vi "FRIC_navX_Internal_USB_ProcessingLoop.vi"(7 "Device Number":T3, 10 "Serial Port":T2=enum."USB 1", 11 "Rate (4Hz-200Hz)":u8=50 min=4 max=200) -> ()   [LabVIEW 2016]
doc: "This navX VI handles the reading/writing for the navX. All of the good stuff is in here.\nTHIS VI SHOULD NOT BE CALLED BY THE USER!"
uses:
  <vilib>/Rock Robotics/SystemInterfaces/i2clib/i2c_bus.ctl
  TypeDefs/Z900_navX_ProtocolTypeDef.ctl
  navX Library v2.lvlib
  TypeDefs/FRIC_navX_ProcessingLoopStatesTypeDef_I2C.ctl
  TypeDefs/Z900_navX_IntegrationControlRegisters.ctl
  TypeDefs/Z900_navX_ActionTypeDef.ctl
  TypeDefs/Z900_navX_NotifyPacketTypeDef.ctl
  TypeDefs/FRIC_navX_I2C Process Loop TypeDef.ctl
  <vilib>/Rock Robotics/SystemInterfaces/spilib/spi_bus.ctl
  <vilib>/Rock Robotics/WPI/SPI/WPI_SPIDevRef.ctl
  TypeDefs/Z900_navX_SerialStreamTypeDef.ctl
  <vilib>/Rock Robotics/WPI/SerialPort/WPI_SerialPortRef.ctl
  TypeDefs/FRIC_navX_DeviceNumbersTypeDef.ctl
  <vilib>/Rock Robotics/WPI/SerialPort/WPI_SerialPort.ctl
  <vilib>/Platform/TimedLoop/XDataNode/wakeup.ctl
  <vilib>/Platform/TimedLoop/XDataNode/XDNodeRunTimeDep.lvlib
  <vilib>/Platform/TimedLoop/XDataNode/nitl_modes.ctl
  <vilib>/Platform/TimedLoop/XDataNode/timing_clust.ctl
  <vilib>/Platform/TimedLoop/XDataNode/XDataNode.xnode
  <vilib>/ptbypt/NI_PtbyPt.lvlib
  TypeDefs/Z900_navX_DeviceTypeDef.ctl
panel:
  in  "Tab Control":enum32{"Page 1", "Page 2"}(tab)
  in  "Halt":bool
  out "Connected 2":bool
  out "error":errorcluster
  in  "Stream Type":T1=enum."AHRSAndPositioning"
  out "Loop Time":dbl format="%#.1g"
  out "Loop dt":i64
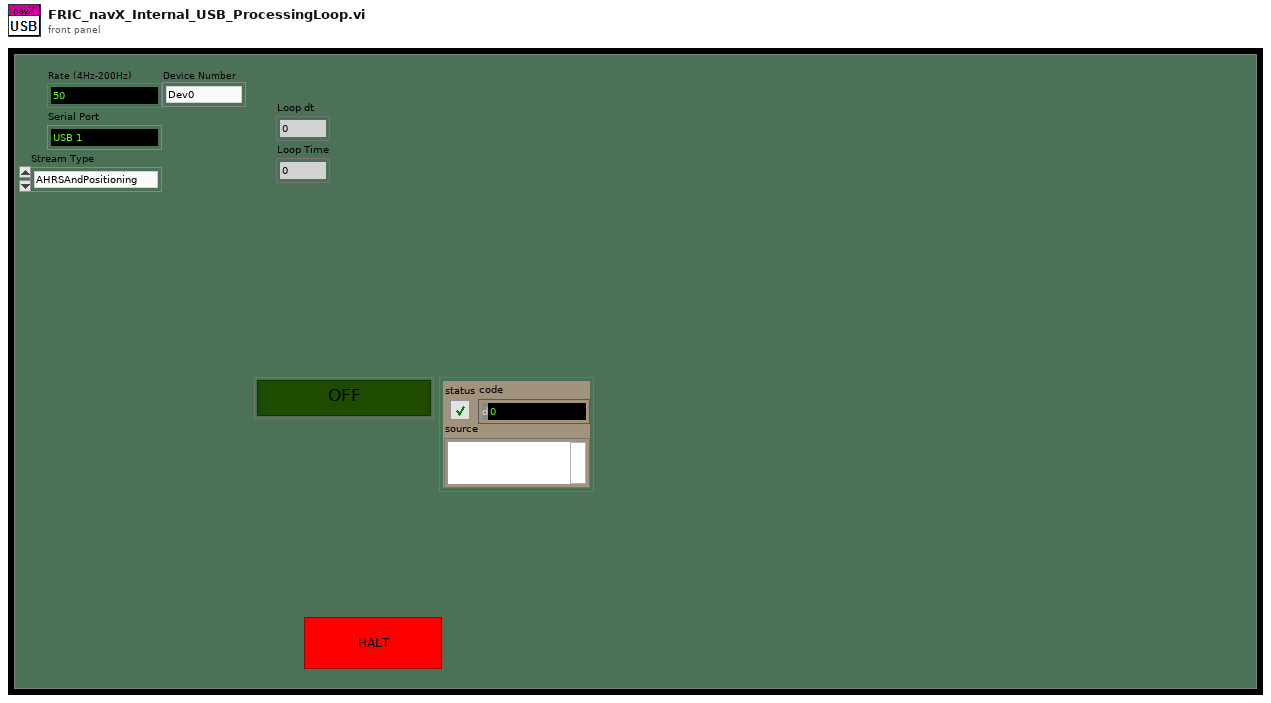
[diagram p1: front panel]
types:
  T1 = typedef "navX Library v2.lvlib/Z900_navX_SerialStreamTypeDef.ctl" = enum16{"YRPH", "Quaterinons", "Gyro/Raw", "AHRS", "AHRSAndPositioning"}
  T2 = typedef "WPI_SerialPort.ctl" = enum16{"Onboard RS-232", "MXP TTL", "USB 1", "USB 2"}
  T3 = typedef "FRIC_navX_DeviceNumbersTypeDef.ctl" = enum16{"Dev0", "Dev1", "Dev2", "Dev3"}
  T4 = typedef "FRIC_navX_I2C Process Loop TypeDef.ctl" = cluster{"State Array":T5[], "error":errorcluster, "FPGA Cluster":cluster{"Last Valid FPGA Time":dbl, "Error Count":i32, "Initialized":bool}, "Device Info":T6, "I2CDevRef":cluster{"DevStatus":errorcluster, "Device Address":u8, "Handle":i32, "I2C Bus":T8}, "Registry":u8[], "Command Array":T9[], "Connected?":bool, "navX Device Memory Size":i32, "notification":T10, "Memory Size Set":bool, "SPIDevRef":T12, "navX Serial Open":cluster{"Stream Type":T1, "Serial Port":T2}, "SerialPortRef":T14, "Serial Read Buffer":string, "Serial Write Buffer":string[], "Device Number":T3, "navX SPI Open":cluster{"SPI Bus":T13, "Clock Rate (Hz)":dbl}, "Loop dt":i64, "current time":timestamp, "Loop Time":i64}
  T5 = typedef "FRIC_navX_ProcessingLoopStatesTypeDef_I2C.ctl" = enum16{"Process", "INI", "Check Packets Valid", "Close", "Flush Serial", "Generate Command", "Last Packet Valid", "Open", "Read", "Reset Serial", "Set Termination Char", "Update AE", "Wait", "Write", "Exit"}
  T6 = typedef "navX Library v2.lvlib/Z900_navX_DeviceTypeDef.ctl" = cluster{"Interface":cluster{"Protocol":T7, "Update Rate (4Hz-100Hz)":u8, "navX Open TypeDef":variant}, "Notify Packet":refnum<notifier>, "Loop VI Refnum":refnum<vi>, "Ready to Close Occurrence Refnum":refnum<k4>}
  T7 = typedef "navX Library v2.lvlib/Z900_navX_ProtocolTypeDef.ctl" = enum16{"SERIAL", "I2C", "SPI"}
  T8 = typedef "i2c_bus.ctl" = enum16{"I2C On-Board", "I2C MXP", "Invalid"}
  T9 = typedef "navX Library v2.lvlib/Z900_navX_IntegrationControlRegisters.ctl" = u8
  T10 = typedef "navX Library v2.lvlib/Z900_navX_NotifyPacketTypeDef.ctl" = cluster{"navX Action":T11, "Data":variant}
  T11 = typedef "navX Library v2.lvlib/Z900_navX_ActionTypeDef.ctl" = enum16{"None", "Halt", "Update Serial Protocol", "Zero-Yaw", "Zero-Displacement", "Zero-Velocity"}
  T12 = typedef "WPI_SPIDevRef.ctl" = cluster{"DevStatus":errorcluster, "Handle":i32, "SPI Bus":T13}
  T13 = typedef "spi_bus.ctl" = enum16{"SPI On-Board, CS0", "SPI On-Board, CS1", "SPI On-Board, CS2", "SPI On-Board, CS3", "SPI MXP", "Invalid"}
  T14 = typedef "WPI_SerialPortRef.ctl" = cluster{"DevStatus":errorcluster, "Serial Port Name":refnum<visa-resource-name>}
  T15 = typedef "XDNodeRunTimeDep.lvlib/timing_clust.ctl" = cluster{"Expected End [f-1]":u64, "Actual End [f-1]":u64, "Finished Late? [f-1]":bool, "Expected End [i-1]":u64, "Actual End [i-1]":u64, "Finished Late? [i-1]":bool, "Expected Start [i]":u64, "Actual Start [i]":u64, "Expected Start [f]":u64, "Actual Start [f]":u64, "Source Name":string, "Structure Name":string, "Period":i64, "Deadline":i64, "Offset":i64, "Start":i64, "Priority":i32, "Timeout":i32, "Mode":T16, "Wakeup Reason":T17, "Error":errorcluster, "Source Type":string, "Secondary Source Type":string, "Global End Time":u64, "Global Start Time":u64, "Frame Duration":u64, "Iteration Duration":u64, "Assigned CPU":i32, "I/O Scan Engine Mode":u32}
  T16 = typedef "XDNodeRunTimeDep.lvlib/nitl_modes.ctl" = enum32{"No Change", "Process missed periods, maintain original phase", "Discard missed periods, maintain original phase", "Process missed periods, ignore original phase", "Discard missed periods, ignore original phase"}
  T17 = typedef "XDNodeRunTimeDep.lvlib/wakeup.ctl" = enum32{"Normal", "Aborted", "Asynchronous wakeup", "Timing source error", "Timed loop error", "Timeout"}
  T18 = typedef "Z900_navX_ActionTypeDef.ctl" = enum16{"None", "Halt", "Normal Read", "Update Serial Protocol", "Update Rate Htz", "Zero-Yaw", "Zero-Displacement", "Zero-Velocity"}
  T19 = cluster{"Last Valid FPGA Time":dbl, "Error Count":i32, "Initialized":bool}
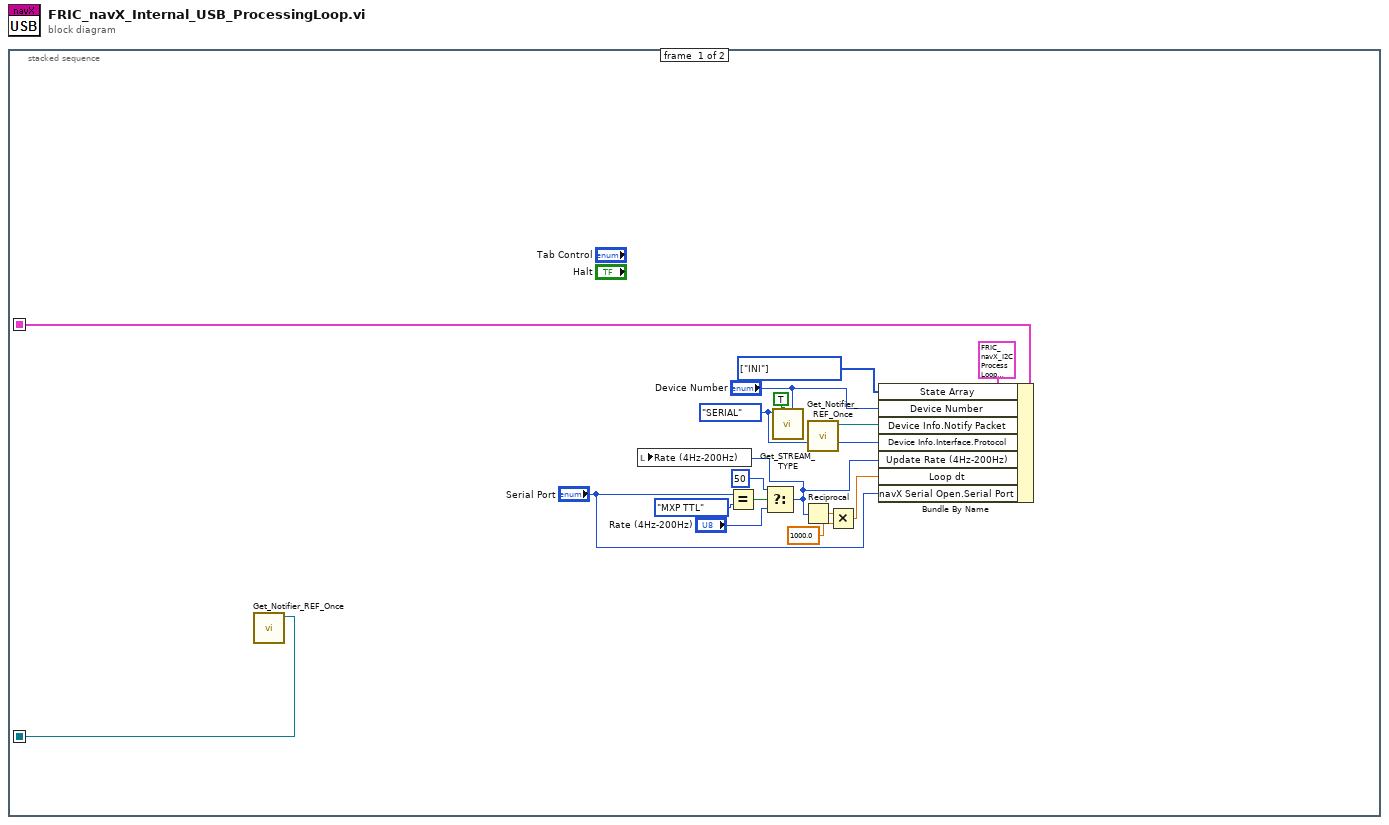
[diagram p0: block diagram]
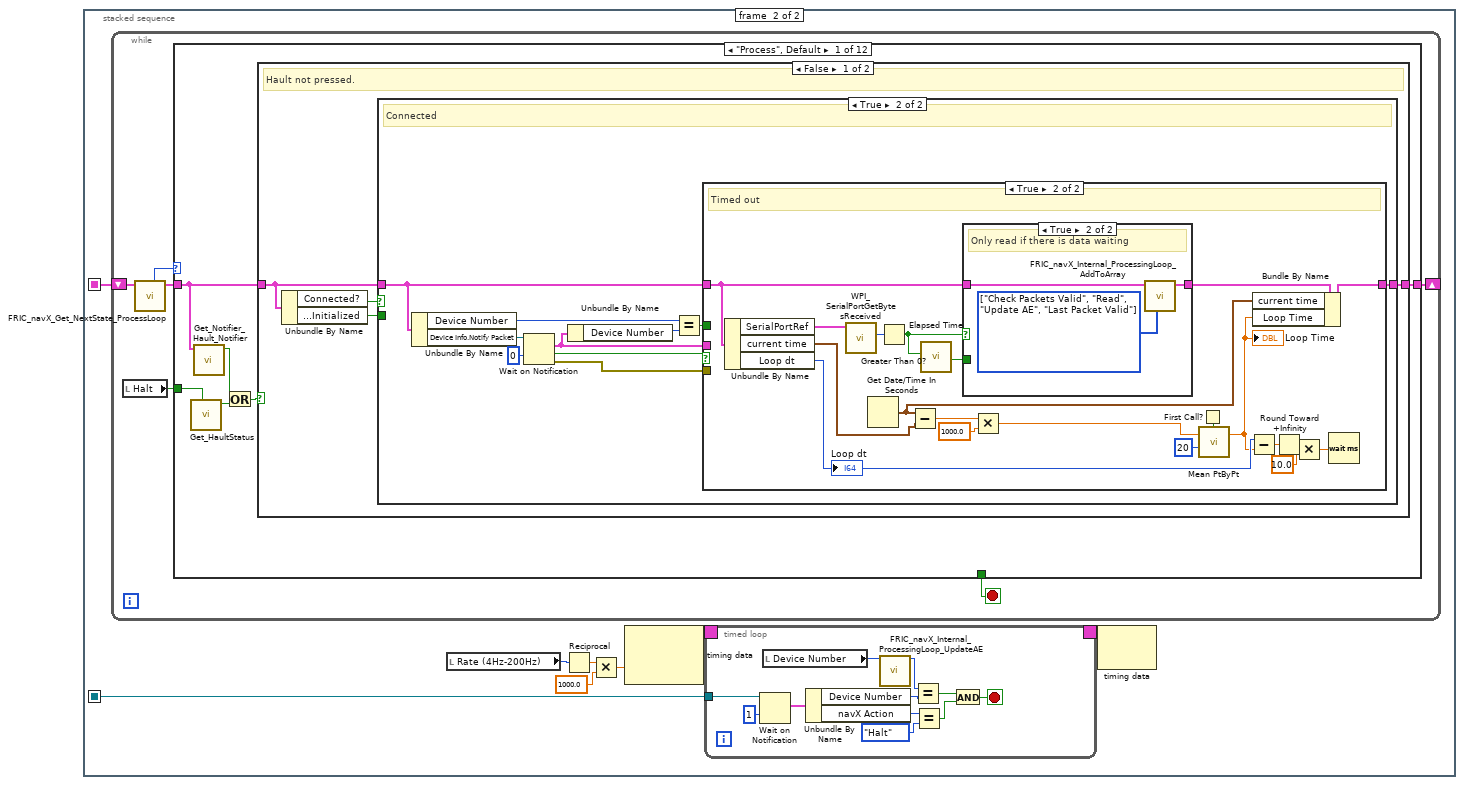
[diagram p2: hidden frame]
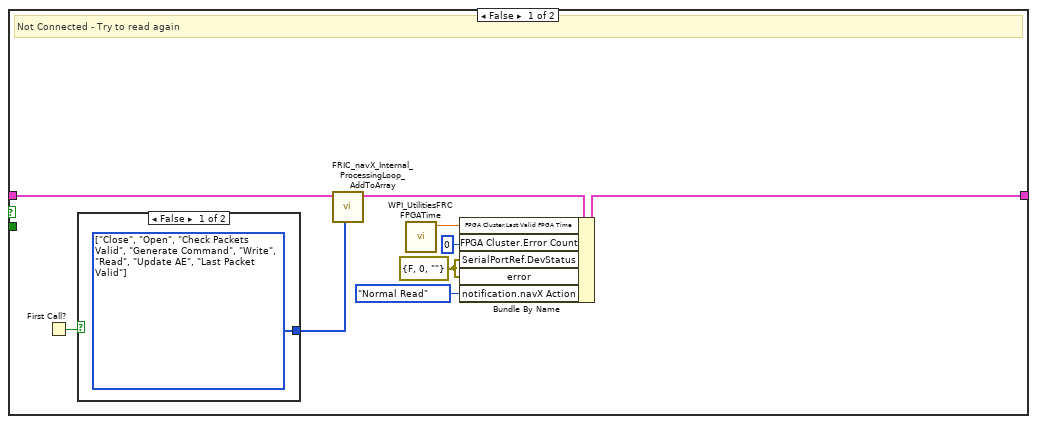
[diagram p3: hidden frame]
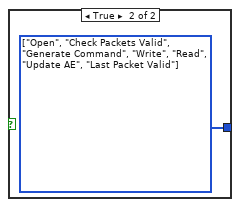
[diagram p4: hidden frame]
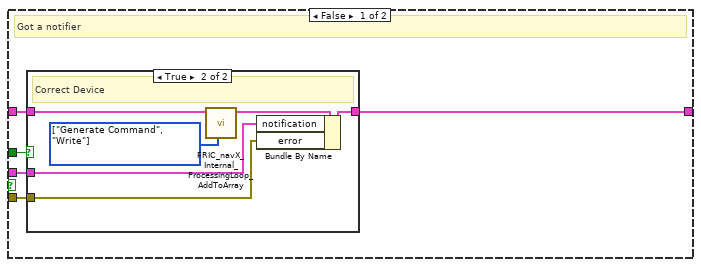
[diagram p5: hidden frame]
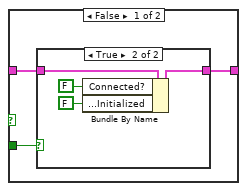
[diagram p7: hidden frame]
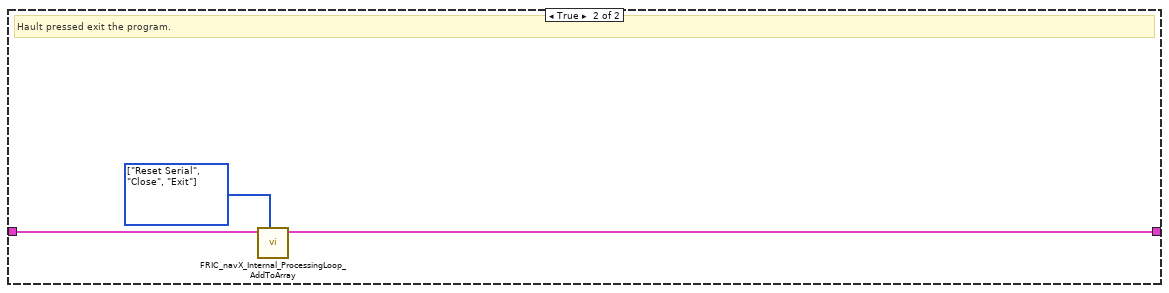
[diagram p9: hidden frame]
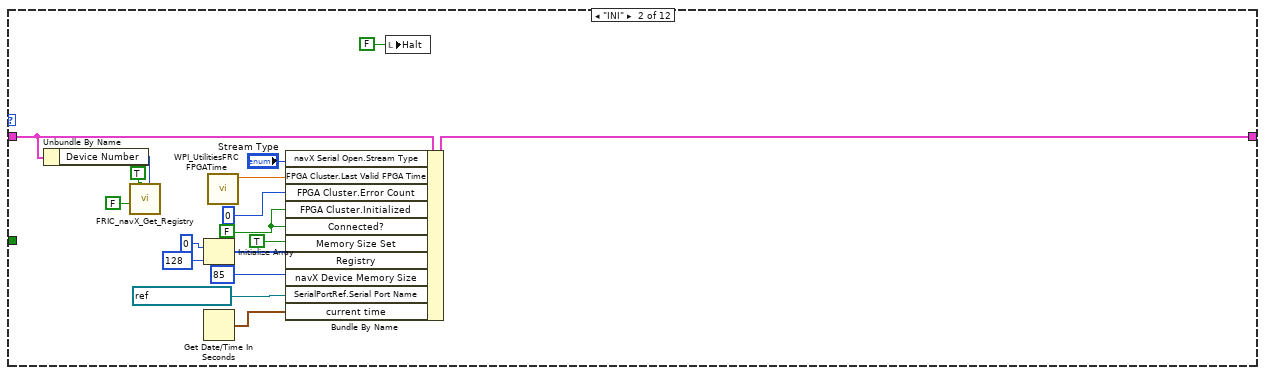
[diagram p10: hidden frame]
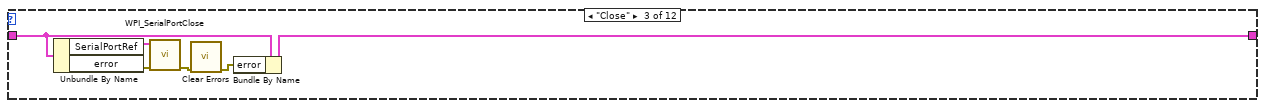
[diagram p11: hidden frame]
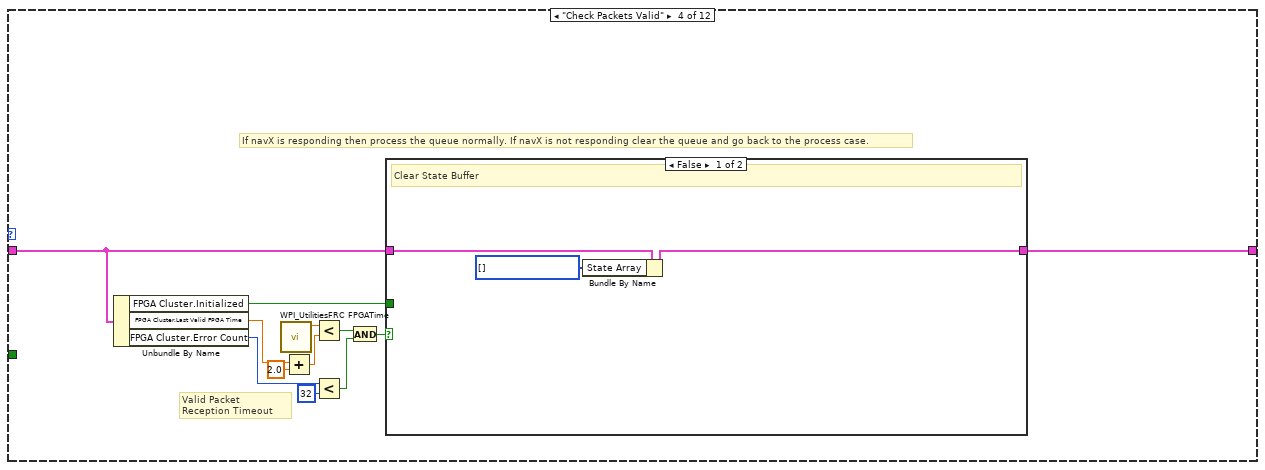
[diagram p12: hidden frame]
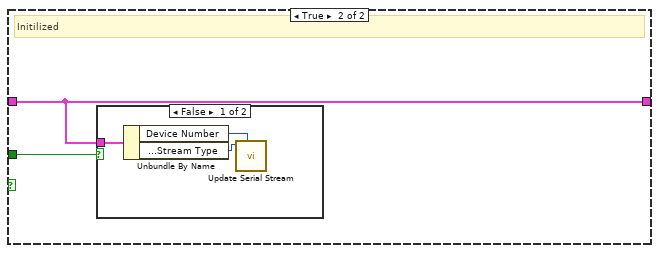
[diagram p13: hidden frame]
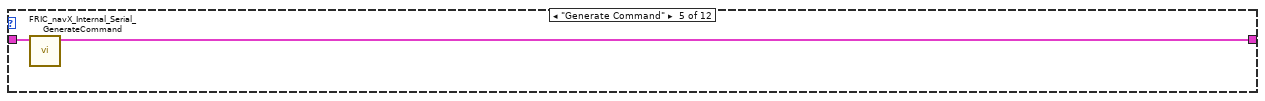
[diagram p15: hidden frame]
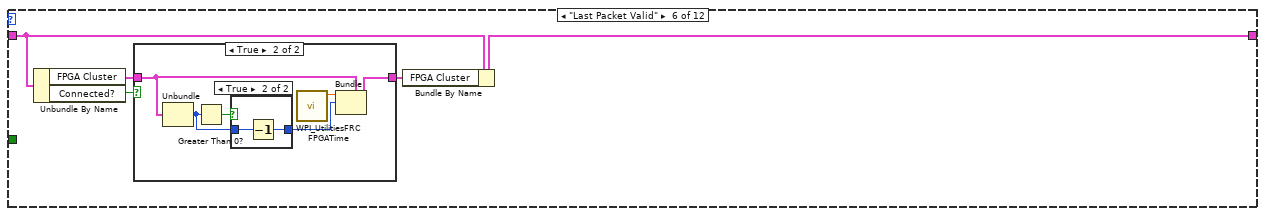
[diagram p16: hidden frame]
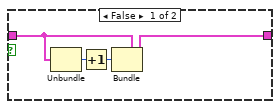
[diagram p17: hidden frame]
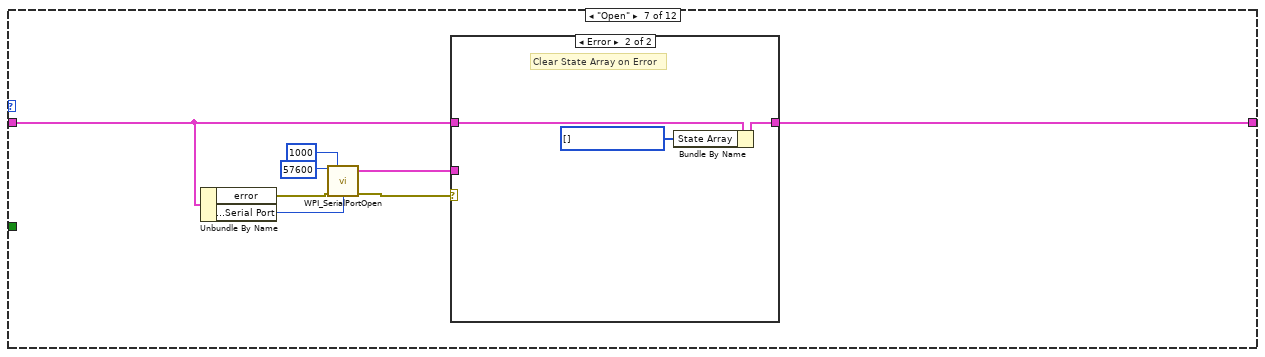
[diagram p19: hidden frame]
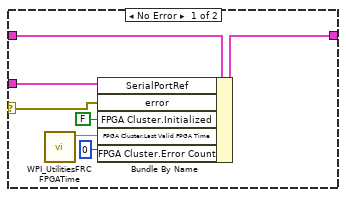
[diagram p20: hidden frame]
diagram:
  n1 = stacked-sequence {
    seq-local: [w17 _] -> [_ w25]
    seq-local: [w13 _] -> [_ w18]
    frame #0 {
      w1 = Z900_navX_ProtocolTypeDef."SERIAL" ("Protocol")
      w15 = T5[] [enum."INI"] items=["Process", "INI", "Check Packets Valid", "Close", "Flush Serial", "Generate Command", "Last Packet Valid", "Open", "Read", "Reset Serial", "Set Termination Char", "Update AE", "Wait", "Write", "Exit"] ("State Array")
      n2 = call "Get_Notifier_REF_Once.vi"() -> ("notifier ref out"=w13:refnum<notifier>)  [unwired: 10 in, 1 out]
      n3 = Equal?(x="Serial Port", y=WPI_SerialPort."MXP TTL") -> (x = y?=w9:bool)
      n4 = Select(t=u8 50, s=w9, f="Rate (4Hz-200Hz)") -> (s? t:f=w4:u8)
      n5 = local write "Rate (4Hz-200Hz)"(w4) -> ()
      n6 = call "Get_STREAM_TYPE.vi"("Device Number"="Device Number", "Update"=TRUE, "Protocol (in)"=w1) -> ()  [unwired: 8 in, 1 out]
      n7 = Reciprocal(x=w4) -> (1/x=w11:dbl)
      n8 = call "Get_Notifier_REF_Once.vi"() -> ("notifier ref out"=w14:refnum<notifier>)  [unwired: 10 in, 1 out]
      n9 = Multiply(x=w11, y=1000.0) -> (x*y=w6:dbl)
      n10 = Bundle By Name(cluster=T4 {"State Array"=[enum."INI", enum."Open"], "error"={"status"=FALSE, "code"=0, "source"=""}, "FPGA Cluster"={"Last Valid FPGA Time"=0.0, "Error Count"=0, "Initialized"=FALSE}, "Device Info"={"Interface"={"Protocol"=enum."SERIAL", "Update Rate (4Hz-100Hz)"=4, "navX Open TypeDef"=variant}, "Notify Packet"=refnum, "Loop VI Refnum"=refnum, "Ready to Close Occurrence Refnum"=refnum}, "I2CDevRef"={"DevStatus"={"status"=FALSE, "code"=0, "source"=""}, "Device Address"=0, "Handle"=0, "I2C Bus"=enum."Invalid"}, "Registry"=[], "Command Array"=[214, 32], "Connected?"=FALSE, "navX Device Memory Size"=85, "notification"={"navX Action"=enum."None", "Data"=variant}, "Memory Size Set"=FALSE, "SPIDevRef"={"DevStatus"={"status"=FALSE, "code"=0, "source"=""}, "Handle"=0, "SPI Bus"=enum."SPI On-Board, CS0"}, "navX Serial Open"={"Stream Type"=enum."YRPH", "Serial Port"=enum."Onboard RS-232"}, "SerialPortRef"={"DevStatus"={"status"=FALSE, "code"=0, "source"=""}, "Serial Port Name"=""}, "Serial Read Buffer"="", "Serial Write Buffer"=[], "Device Number"=enum."Dev0", "navX SPI Open"={"SPI Bus"=enum."SPI MXP", "Clock Rate (Hz)"=500000.0}, "Loop dt"=0, "current time"=timestamp(0 s since 1904-01-01), "Loop Time"=0} ("I2C Process Loop TypeDef"), "State Array"=w15, "Device Number"="Device Number", "Device Info.Notify Packet"=w14, "Device Info.Interface.Protocol"=w1, "Update Rate (4Hz-200Hz)"=w4, "Loop dt"=w6, "navX Serial Open.Serial Port"="Serial Port") -> (w17:T4)
    }
    frame #1 {
      n11 = while {
        shift-right: [w43] -> _
        shift-left: w25 -> [w46]
        stop <- w47 stop-if-true
        n12 = local read "Halt"() -> (w42:bool)
        n13 = call "FRIC_navX_Get_NextState_ProcessLoop.vi"("I2C Process Loop TypeDef (in)"=w46) -> ("I2C Process Loop TypeDef (out)"=w45:T4, "Current State"=w44:T5)  [unwired: 9 in]
        n14 = case shown="\"Process\", Default" w44 {
          tunnel: [_ _ _ _ _ _ _ _ _ _ TRUE _] -> w47
          tunnel: w45 -> [w51 w130 w147 w152 w169 w173 w195 w223 w241 w254 w261 w269]
          tunnel: [w53 w137 w146 w153 w168 w172 w194 w215 w242 w243 w261 w269] -> w43
          tunnel: w42 -> [w52 _ _ _ _ _ _ _ _ _ _ _]
          frame "Process", Default {
            n15 = call "Get_HaultStatus.vi"("Update"=w52) -> ("Hault"=w49:bool)  [unwired: 10 in]
            n16 = call "Get_Notifier_Hault_Notifier.vi"("Process Loop TypeDef (in)"=w51) -> ("Hault Notifier"=w50:bool)  [unwired: 10 in]
            n17 = Or(x=w50, y=w49) -> (x .or. y?=w48:bool)
            n18 = case shown="False" w48 {
              tunnel: [w57 w123] -> w53
              tunnel: w51 -> [w55 w124]
              frame False {
                # "Hault not pressed."
                n19 = Unbundle By Name(w55) -> ("Connected?"=w56:bool, "FPGA Cluster.Initialized"=w54:bool)
                n20 = case shown="True" w56 {
                  tunnel: w55 -> [w66 w69]
                  tunnel: [w63 w78] -> w57
                  tunnel: w54 -> [_ _]
                  frame False {
                    w60 = errorcluster {"status"=FALSE, "code"=0, "source"=""} ("SerialPortRef.DevStatus")
                    # "Not Connected - Try to read again"
                    n21 = First Call?() -> (First Call?: T/F=w59:bool)
                    n22 = case shown="False" w59 {
                      tunnel: [w67 w68] -> w65
                      frame False {
                        w67 = T5[] [enum."Close", enum."Open", enum."Check Packets Valid", enum."Generate Command", enum."Write", enum."Read", enum."Update AE", enum."Last Packet Valid"] items=["Process", "INI", "Check Packets Valid", "Close", "Flush Serial", "Generate Command", "Last Packet Valid", "Open", "Read", "Reset Serial", "Set Termination Char", "Update AE", "Wait", "Write", "Exit"]
                      }
                      frame True {
                        w68 = T5[] [enum."Open", enum."Check Packets Valid", enum."Generate Command", enum."Write", enum."Read", enum."Update AE", enum."Last Packet Valid"] items=["Process", "INI", "Check Packets Valid", "Close", "Flush Serial", "Generate Command", "Last Packet Valid", "Open", "Read", "Reset Serial", "Set Termination Char", "Update AE", "Wait", "Write", "Exit"]
                      }
                    }
                    n23 = call "FRIC_navX_Internal_ProcessingLoop_AddToArray.vi"("States Array"=w65, "I2C Process Loop TypeDef (in)"=w66) -> ("I2C Process Loop TypeDef (out)"=w64:T4)  [unwired: 9 in]
                    n24 = call <vilib>:"WPI_UtilitiesFRC FPGATime.vi"() -> ("FPGA Time"=w61:dbl)  [unwired: 10 in, 1 out]
                    n25 = Bundle By Name(cluster=w64, "FPGA Cluster.Last Valid FPGA Time"=w61, "FPGA Cluster.Error Count"=0, "SerialPortRef.DevStatus"=w60, "error"=w60, "notification.navX Action"=Z900_navX_ActionTypeDef."Normal Read") -> (w63:T4)
                  }
                  frame True {
                    # "Connected"
                    n26 = Unbundle By Name(w69) -> ("Device Number"=w72:T3, "Device Info.Notify Packet"=w77:refnum<notifier>)
                    n27 = Wait on Notification(notifier=w77, timeout in ms (-1)=0) -> (notification=w73:T10, timed out?=w74:bool, error out=w75:errorcluster)  [unwired: 2 in, 1 out]
                    n28 = Unbundle By Name(w73) -> ("Device Number"=w71:T3)
                    n29 = Equal?(x=w72, y=w71) -> (x = y?=w70:bool)
                    n30 = case shown="True" w74 {
                      tunnel: w69 -> [w83 w107]
                      tunnel: [w82 w104] -> w78
                      tunnel: w73 -> [w81 _]
                      tunnel: w75 -> [w80 _]
                      tunnel: w70 -> [w79 _]
                      frame False {
                        # "Got a notifier"
                        n31 = case shown="True" w79 {
                          tunnel: w83 -> [w84 w90]
                          tunnel: [w84 w89] -> w82
                          tunnel: w81 -> [_ w88]
                          tunnel: w80 -> [_ w85]
                          frame False {
                          }
                          frame True {
                            w86 = T5[] [enum."Generate Command", enum."Write"] items=["Process", "INI", "Check Packets Valid", "Close", "Flush Serial", "Generate Command", "Last Packet Valid", "Open", "Read", "Reset Serial", "Set Termination Char", "Update AE", "Wait", "Write", "Exit"] ("States Array")
                            # "Correct Device"
                            n32 = call "FRIC_navX_Internal_ProcessingLoop_AddToArray.vi"("States Array"=w86, "I2C Process Loop TypeDef (in)"=w90) -> ("I2C Process Loop TypeDef (out)"=w87:T4)  [unwired: 9 in]
                            n33 = Bundle By Name(cluster=w87, "notification"=w88, "error"=w85) -> (w89:T4)
                          }
                        }
                      }
                      frame True {
                        # "Timed out"
                        n34 = Unbundle By Name(w107) -> ("SerialPortRef"=w109:T14, "current time"=w103:timestamp, "Loop dt"=w92:i64)
                        "Loop dt" <- w92
                        n35 = call <vilib>:"WPI_SerialPortGetBytesReceived.vi"("SerialPortRef"=w109) -> ("Bytes at Port"=w108:u32)  [unwired: 8 in, 2 out]
                        n36 = Get Date/Time In Seconds() -> (seconds since 1Jan1904=w102:timestamp)
                        n37 = Greater Than 0?(x=w108) -> (x > 0?=w106:bool)
                        n38 = Subtract(x=w102, y=w103) -> (x-y=w101:dbl)
                        n39 = call "Elapsed Time"("Reset"=w106) -> ("Time has Elapsed"=w105:bool)  [unwired: 11 in, 7 out]
                        n40 = case shown="True" w106 {
                          tunnel: [w112 w120] -> w110
                          tunnel: w107 -> [w113 w119]
                          tunnel: w105 -> [w111 _]
                          frame False {
                            n41 = case shown="True" w111 {
                              tunnel: w113 -> [w114 w118]
                              tunnel: [w114 w117] -> w112
                              frame False {
                              }
                              frame True {
                                n42 = Bundle By Name(cluster=w118, "Connected?"=FALSE, "FPGA Cluster.Initialized"=FALSE) -> (w117:T4)
                              }
                            }
                          }
                          frame True {
                            w121 = T5[] [enum."Check Packets Valid", enum."Read", enum."Update AE", enum."Last Packet Valid"] items=["Process", "INI", "Check Packets Valid", "Close", "Flush Serial", "Generate Command", "Last Packet Valid", "Open", "Read", "Reset Serial", "Set Termination Char", "Update AE", "Wait", "Write", "Exit"]
                            # "Only read if there is data waiting"
                            n43 = call "FRIC_navX_Internal_ProcessingLoop_AddToArray.vi"("States Array"=w121, "I2C Process Loop TypeDef (in)"=w119) -> ("I2C Process Loop TypeDef (out)"=w120:T4)  [unwired: 9 in]
                          }
                        }
                        n44 = Multiply(x=w101, y=1000.0) -> (x*y=w93:dbl)
                        n45 = First Call?() -> (First Call?: T/F=w95:bool)
                        n46 = call <vilib>:"Mean PtByPt.vi"("x"=w93, "sample length"=20, "initialize"=w95) -> ("mean"=w91:dbl)  [unwired: 1 in, 1 out]
                        "Loop Time" <- w91
                        n47 = Subtract(x=w92, y=w91) -> (x-y=w97:dbl)
                        n48 = Bundle By Name(cluster=w110, "current time"=w102, "Loop Time"=w91) -> (w104:T4)
                        n49 = Round Toward +Infinity(x=w97) -> (ceil(x): smallest int >= x=w99:dbl)
                        n50 = Multiply(x=w99, y=10.0) -> (x*y=w94:dbl)
                        n51 = Wait (ms)(milliseconds to wait=w94) -> ()  [unwired: 1 out]
                      }
                    }
                  }
                }
              }
              frame True {
                w122 = T5[] [enum."Reset Serial", enum."Close", enum."Exit"] items=["Process", "INI", "Check Packets Valid", "Close", "Flush Serial", "Generate Command", "Last Packet Valid", "Open", "Read", "Reset Serial", "Set Termination Char", "Update AE", "Wait", "Write", "Exit"] ("States Array")
                # "Hault pressed exit the program."
                n52 = call "FRIC_navX_Internal_ProcessingLoop_AddToArray.vi"("States Array"=w122, "I2C Process Loop TypeDef (in)"=w124) -> ("I2C Process Loop TypeDef (out)"=w123:T4)  [unwired: 9 in]
              }
            }
          }
          frame "INI" {
            w135 = FALSE ("Initialized")
            n53 = Unbundle By Name(w130) -> ("Device Number"=w129:T3)
            n54 = call "FRIC_navX_Get_Registry.vi"("Device Number"=w129, "Update"=TRUE, "Connected?"=FALSE) -> ()  [unwired: 7 in, 2 out]
            n55 = Initialize Array(u8 0 ("Received Data"), 128 ("hex")) -> (w133:u8[])
            n56 = Get Date/Time In Seconds() -> (seconds since 1Jan1904=w125:timestamp)
            n57 = call <vilib>:"WPI_UtilitiesFRC FPGATime.vi"() -> ("FPGA Time"=w139:dbl)  [unwired: 10 in, 1 out]
            n58 = Bundle By Name(cluster=w130, "navX Serial Open.Stream Type"="Stream Type", "FPGA Cluster.Last Valid FPGA Time"=w139, "FPGA Cluster.Error Count"=0 ("Error Count"), "FPGA Cluster.Initialized"=w135, "Connected?"=w135, "Memory Size Set"=TRUE, "Registry"=w133, "navX Device Memory Size"=85 ("hex"), "SerialPortRef.Serial Port Name"=refnum<visa-resource-name> "ASRL3::INSTR" ("Serial Port Name"), "current time"=w125) -> (w137:T4)
            n59 = local write "Halt"(FALSE ("Halt")) -> ()
          }
          frame "Close" {
            n60 = Unbundle By Name(w147) -> ("SerialPortRef"=w144:T14, "error"=w143:errorcluster)
            n61 = call <vilib>:"WPI_SerialPortClose.vi"("error in (no error)"=w143, "SerialPortRef"=w144) -> ("error out"=w142:errorcluster)  [unwired: 9 in]
            n62 = call <vilib>:"Clear Errors.vi"("error in (no error)"=w142) -> ("error out"=w145:errorcluster)  [unwired: 5 in, 1 out]
            n63 = Bundle By Name(cluster=w147, "error"=w145) -> (w146:T4)
          }
          frame "Check Packets Valid" {
            # "If navX is responding then process the queue normally. If navX is not responding clear the queue and go back to the process case."
            # "Valid Packet Reception Timeout"
            n64 = Unbundle By Name(w152) -> ("FPGA Cluster.Initialized"=w148:bool, "FPGA Cluster.Last Valid FPGA Time"=w151:dbl, "FPGA Cluster.Error Count"=w150:i32)
            n65 = call <vilib>:"WPI_UtilitiesFRC FPGATime.vi"() -> ("FPGA Time"=w157:dbl)  [unwired: 10 in, 1 out]
            n66 = Add(x=w151, y=2.0) -> (x+y=w158:dbl)
            n67 = Less?(x=w157, y=w158) -> (x < y?=w155:bool)
            n68 = Less?(x=w150, y=32) -> (x < y?=w154:bool)
            n69 = And(x=w155, y=w154) -> (x .and. y?=w149:bool)
            n70 = case shown="False" w149 {
              tunnel: w152 -> [w162 w164]
              tunnel: [w161 w164] -> w153
              tunnel: w148 -> [_ w163]
              frame False {
                w160 = T5[] [] items=["Process", "INI", "Check Packets Valid", "Close", "Flush Serial", "Generate Command", "Last Packet Valid", "Open", "Read", "Reset Serial", "Set Termination Char", "Update AE", "Wait", "Write", "Exit"] ("f")
                # "Clear State Buffer"
                n71 = Bundle By Name(cluster=w162, "State Array"=w160) -> (w161:T4)
              }
              frame True {
                # "Initilized"
                n72 = case shown="False" w163 {
                  tunnel: w164 -> [w165 _]
                  frame False {
                    n73 = Unbundle By Name(w165) -> ("Device Number"=w166:T3, "navX Serial Open.Stream Type"=w167:T1)
                    n74 = call "Update Serial Stream.vi"("Device Number"=w166, "Stream Type"=w167) -> ()  [unwired: 10 in]
                  }
                  frame True {
                  }
                }
              }
            }
          }
          frame "Generate Command" {
            n75 = call "FRIC_navX_Internal_Serial_GenerateCommand.vi"("Serial Process Loop TypeDef (in)"=w169) -> ("Serial Process Loop TypeDef (out)"=w168:T4)  [unwired: 10 in]
          }
          frame "Last Packet Valid" {
            n76 = Unbundle By Name(w173) -> ("FPGA Cluster"=w174:T19, "Connected?"=w170:bool)
            n77 = case shown="True" w170 {
              tunnel: [w177 w184] -> w171
              tunnel: w174 -> [w176 w180]
              frame False {
                n78 = Unbundle(w176) -> ("Error Count"=w175:i32)  [unwired: 2 out]
                n79 = Increment(x=w175) -> (x+1=w178:i32)
                n80 = Bundle(cluster=w176, "Error Count"=w178) -> (w177:T19)  [unwired: 2 in]
              }
              frame True {
                n81 = Unbundle(w180) -> ("Error Count"=w179:i32)  [unwired: 2 out]
                n82 = Greater Than 0?(x=w179) -> (x > 0?=w182:bool)
                n83 = case shown="True" w182 {
                  tunnel: [w185 w187] -> w181
                  tunnel: w179 -> [w185 w186]
                  frame False {
                  }
                  frame True {
                    n84 = Decrement(x=w186) -> (x-1=w187:i32)
                  }
                }
                n85 = call <vilib>:"WPI_UtilitiesFRC FPGATime.vi"() -> ("FPGA Time"=w183:dbl)  [unwired: 10 in, 1 out]
                n86 = Bundle(cluster=w180, "Last Valid FPGA Time"=w183, "Error Count"=w181) -> (w184:T19)  [unwired: 1 in]
              }
            }
            n87 = Bundle By Name(cluster=w173, "FPGA Cluster"=w171) -> (w172:T4)
          }
          frame "Open" {
            n88 = Unbundle By Name(w195) -> ("error"=w191:errorcluster, "navX Serial Open.Serial Port"=w188:T2)
            n89 = call <vilib>:"WPI_SerialPortOpen.vi"("Baud Rate"=u32 57600, "Timeout Value (ms)"=u32 1000, "error in (no error)"=w191, "Serial Port"=w188) -> ("SerialPortRef"=w193:T14, "error out"=w192:errorcluster)  [unwired: 10 in]
            n90 = case shown="Error" w192 {
              selector: w192 -> [w196 _]
              tunnel: w195 -> [w202 w205]
              tunnel: [w201 w204] -> w194
              tunnel: w193 -> [w199 _]
              frame No Error {
                n91 = call <vilib>:"WPI_UtilitiesFRC FPGATime.vi"() -> ("FPGA Time"=w198:dbl)  [unwired: 10 in, 1 out]
                n92 = Bundle By Name(cluster=w202, "SerialPortRef"=w199, "error"=w196, "FPGA Cluster.Initialized"=FALSE ("Initialized"), "FPGA Cluster.Last Valid FPGA Time"=w198, "FPGA Cluster.Error Count"=0) -> (w201:T4)
              }
              frame Error {
                w203 = T5[] [] items=["Process", "INI", "Check Packets Valid", "Close", "Flush Serial", "Generate Command", "Last Packet Valid", "Open", "Read", "Reset Serial", "Set Termination Char", "Update AE", "Wait", "Write", "Exit"] ("State Array")
                # "Clear State Array on Error"
                n93 = Bundle By Name(cluster=w205, "State Array"=w203) -> (w204:T4)
              }
            }
          }
          frame "Read" {
            n94 = Unbundle By Name(w223) -> ("Serial Read Buffer"=w228:string, "SerialPortRef"=w229:T14, "SerialPortRef.Serial Port Name"=w231:refnum<visa-resource-name>, "error"=w230:errorcluster, "Device Number"=w208:T3, "Registry"=w224:u8[])
            n95 = property class="Instr"(reference=w231, error in=w230) -> (error out=w225:errorcluster, "Bytes at Port"=w212:u32)  [unwired: 1 in]
            n96 = Greater?(x=w212, y=u32 512) -> (0:w214:bool)
            n97 = Select(t=u32 512 ("y"), s=w214, f=w212) -> (s? t:f=w211:u32)
            n98 = call <vilib>:"WPI_SerialPortRead.vi"("error in (no error)"=w225, "Num Bytes to Read"=w211, "SerialPortRef"=w229) -> ("error out"=w207:errorcluster, "Buffer"=w222:string)  [unwired: 6 in, 1 out]
            n99 = call "FRIC_navX_Clear_Buffer_Warning.vi"("error in"=w207) -> ("error out"=w206:errorcluster)  [unwired: 10 in]
            n100 = Concatenate Strings(w228, w222) -> (w221:string)
            n101 = Not(x=w206) -> (.not. x?=w213:bool)
            "Connected 2" <- w213
            n102 = call "Z900_navX_SERIAL_CapturePacket.vi"("Buffer"=w221) -> ("Packet"=w218:string, "Buffer"=w220:string)  [unwired: 7 in, 2 out]
            n103 = call "Z900_navX_SERIAL_DecodePacket.vi"("Data"=w224, "Packet"=w218) -> (1:w210, "Data"=w219:u8[])  [unwired: 6 in, 2 out]
            n104 = Not(x=w210) -> (.not. x?=w209:bool)
            n105 = call "FRIC_navX_Get_Registry.vi"("Device Number"=w208, "Update"=w209, "Connected?"=w213, "Registry (in)"=w219) -> ()  [unwired: 6 in, 2 out]
            n106 = Bundle By Name(cluster=w223, "Serial Read Buffer"=w220, "Connected?"=w213, "error"=w206) -> (w216:T4)
            n107 = call "Get_Connect_Status.vi"("Device Number"=w208, "Update"=TRUE, "Connected"=w213) -> ()  [unwired: 8 in, 1 out]
            n108 = case shown="False" w214 {
              tunnel: w216 -> [w232 w236]
              tunnel: [w232 w235] -> w215
              frame False {
              }
              frame True {
                w234 = T5[] [enum."Read"] items=["Process", "INI", "Check Packets Valid", "Close", "Flush Serial", "Generate Command", "Last Packet Valid", "Open", "Read", "Reset Serial", "Set Termination Char", "Update AE", "Wait", "Write", "Exit"] ("States Array")
                n109 = call "FRIC_navX_Internal_ProcessingLoop_AddToArray.vi"("Add to beginning"=TRUE, "States Array"=w234, "I2C Process Loop TypeDef (in)"=w236) -> ("I2C Process Loop TypeDef (out)"=w235:T4)  [unwired: 8 in]
              }
            }
          }
          frame "Reset Serial" {
            n110 = Unbundle By Name(w241) -> ("SerialPortRef"=w240:T14, "error"=w238:errorcluster)
            n111 = call <vilib>:"WPI_SerialPortReset.vi"("error in (no error)"=w238, "SerialPortRef"=w240) -> ("error out"=w237:errorcluster, "SerialPortRef"=w239:T14)  [unwired: 8 in]
            n112 = Bundle By Name(cluster=w241, "SerialPortRef"=w239, "error"=w237) -> (w242:T4)
          }
          frame "Write" {
            n113 = Unbundle By Name(w254) -> ("SerialPortRef"=w252:T14, "Serial Write Buffer"=w249:string[], "SerialPortRef.DevStatus"=w253:errorcluster)
            n114 = Delete From Array(array=w249, index=0) -> (deleted portion=w248:string, array with subset deleted=w245:string[])  [unwired: 1 in]
            n115 = call <vilib>:"WPI_SerialPortWrite.vi"("error in (no error)"=w253, "Buffer"=w248, "SerialPortRef"=w252) -> ("error out"=w251:errorcluster, "SerialPortRef"=w250:T14)  [unwired: 6 in, 1 out]
            n116 = Empty Array?(array=w245) -> (empty?=w244:bool)
            n117 = Bundle By Name(cluster=w254, "SerialPortRef"=w250, "error"=w251, "Serial Write Buffer"=w245) -> (w246:T4)
            n118 = case shown="False" w244 {
              tunnel: [w258 w259] -> w243
              tunnel: w246 -> [w257 w259]
              frame False {
                w256 = T5[] [enum."Write"] items=["Process", "INI", "Check Packets Valid", "Close", "Flush Serial", "Generate Command", "Last Packet Valid", "Open", "Read", "Reset Serial", "Set Termination Char", "Update AE", "Wait", "Write", "Exit"] ("States Array")
                # "Write again because buffer is not empty."
                n119 = call "FRIC_navX_Internal_ProcessingLoop_AddToArray.vi"("Add to beginning"=TRUE, "States Array"=w256, "I2C Process Loop TypeDef (in)"=w257) -> ("I2C Process Loop TypeDef (out)"=w258:T4)  [unwired: 8 in]
              }
              frame True {
                # "Process the rest of the state array"
              }
            }
          }
          frame "Exit" {
            n120 = Unbundle By Name(w261) -> ("Device Info"=w260:T6)
            n121 = in-place {
              in-place-border: w260 -> [w264]
              # "Set Occurence of Close"
              n122 = Unbundle By Name(w264) -> ("Ready to Close Occurrence Refnum"=w265:refnum<k4>)
              n123 = local write "Halt"(FALSE ("Halt")) -> ()
              n124 = Set Occurrence(w265) -> ()
            }
          }
          frame "Update AE" {
            n125 = Unbundle By Name(w269) -> ("Device Number"=w266:T3, "error"=w268:errorcluster)
            "error" <- w268
            n126 = call "Get_Error_Status.vi"("Device Number"=w266, "Update"=TRUE, "error in"=w268) -> ()  [unwired: 8 in, 1 out]
          }
        }
      }
      n127 = local read "Rate (4Hz-200Hz)"() -> (w23:u8)
      n128 = Reciprocal(x=w23) -> (1/x=w24:dbl)
      n129 = Multiply(x=w24, y=1000.0) -> (x*y=w19:dbl)
      n130 = node-c288(w19) -> (w21:T15)  [unwired: 1 in]
      n131 = timed-loop {
        timing: w21 -> [_]
        timing-out: [_] -> w20
        tunnel: w18 -> [w32]
        stop <- w26 stop-if-true
        n132 = Wait on Notification(notifier=w32, timeout in ms (-1)=1) -> (notification=w31:T10)  [unwired: 2 in, 3 out]
        n133 = local read "Device Number"() -> (w29:T3)
        n134 = Unbundle By Name(w31) -> ("Device Number"=w30:T3, "navX Action"=w34:T11)
        n135 = call "FRIC_navX_Internal_ProcessingLoop_UpdateAE.vi"("Device Number"=w29) -> ()  [unwired: 15 in]
        n136 = Equal?(x=w29, y=w30) -> (x = y?=w28:bool)
        n137 = Equal?(x=w34, y=Z900_navX_ActionTypeDef."Halt") -> (x = y?=w27:bool)
        n138 = And(x=w28, y=w27) -> (x .and. y?=w26:bool)
      }
      n139 = node-c288(w20) -> ()  [unwired: 1 out]
    }
  }
